vi "GetImageFileMachineVersion.vi"(8 "error in":errorcluster, 11 "dll Path":path) -> (0 "error out":errorcluster, 2 "bitness":enum16{"unknown", "32", "64"}(ring), 3 "path":path)   [LabVIEW 2017]
doc: "This VI can will read the PE Header to read the Machine type (x86 or x64)"
uses:
  <vilib>/ErrorRing/Error Ring.xnode
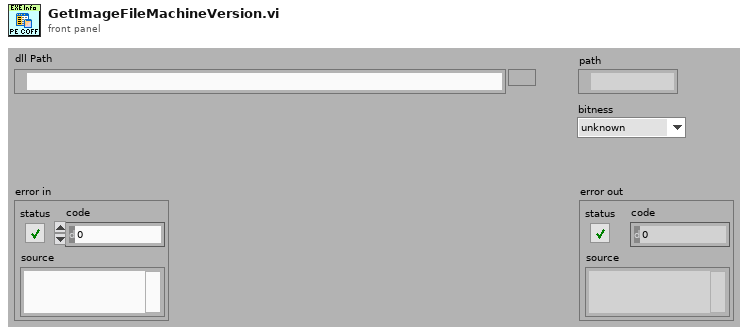
[diagram p1: front panel]
types:
  T1 = enum16{"open", "replace", "create", "open or create", "replace or create", "replace or create with confirmation"}
  T2 = enum16{"big-endian, network order", "native, host order", "little-endian"}
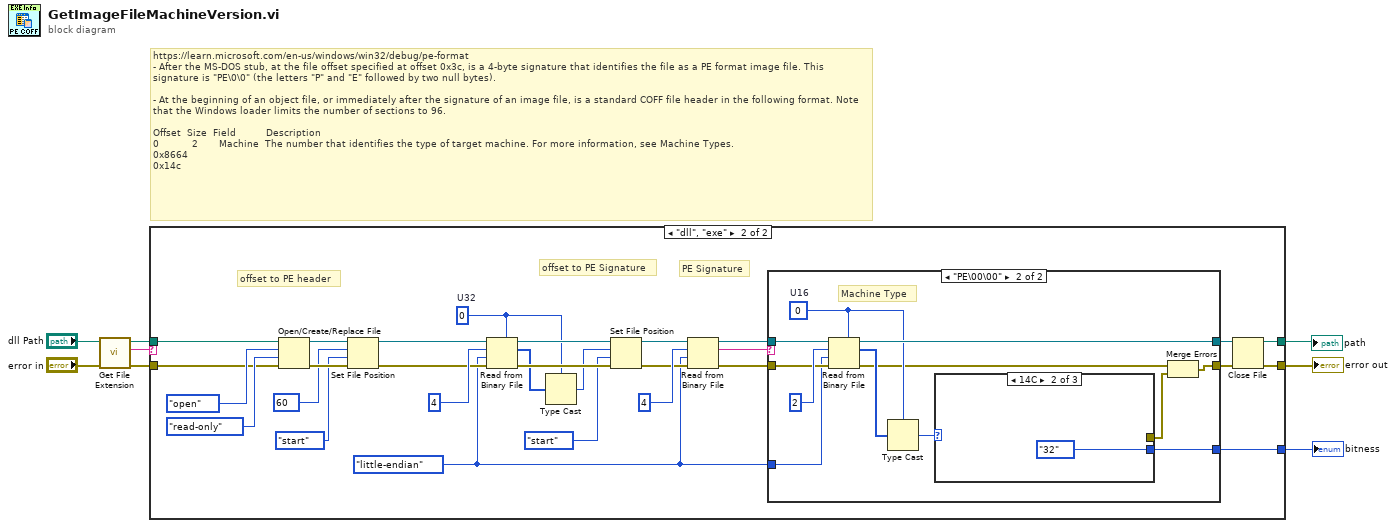
[diagram p0: block diagram]
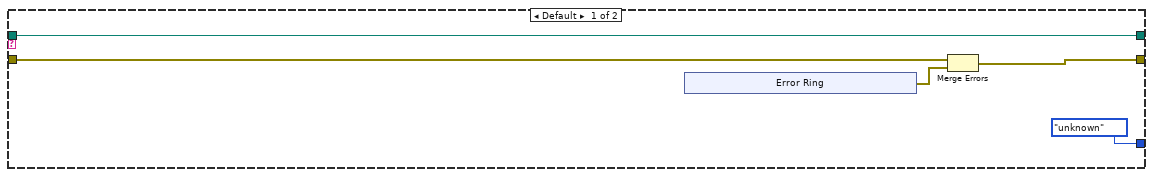
[diagram p2: hidden frame]
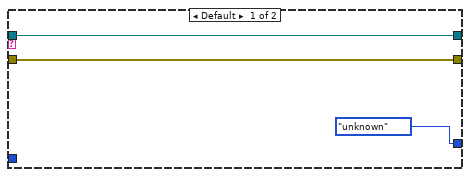
[diagram p3: hidden frame]
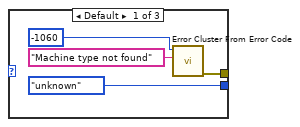
[diagram p4: hidden frame]
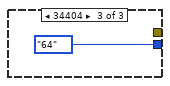
[diagram p5: hidden frame]
diagram:
  # "https://learn.microsoft.com/en-us/windows/win32/debug/pe-format\n- After the MS-DOS stub, at the file offset specified at offset 0x3c, is a 4-byte signature that identifies the file as a PE format image file. This signature is \"PE\\0\\0\" (the letters \"P\" and \"E\" followed by two null bytes).\n\n- At the beginning of an object file, or immediately after the signature of an image file, is a standard COFF file header in the following format. Note that the Windows loader limits the number of sections to 96.\n\nOffset \tSize \tField \t        Description\n0\t          2\t      Machine\t The number that identifies the type of target machine. For more information, see Machine Types. \n0x8664 \n0x14c"
  n1 = call <vilib>:"Get File Extension.vi"("error in (no error)"="error in", "file"="dll Path") -> ("error out"=w6:errorcluster, "lowercase file extension"=w4:string, "dup file"=w5:path)  [unwired: 5 in, 2 out]
  n2 = case shown="\"dll\", \"exe\"" w4 {
    tunnel: w6 -> [w13 w26]
    tunnel: w5 -> [w9 w25]
    tunnel: [w11 w22] -> w3
    tunnel: [enum16{"unknown", "32", "64"}."unknown" ("bitness") w20] -> w2
    tunnel: [w9 w18] -> w1
    frame Default {
      n3 = xnode "Error Ring"() -> ("error out"=w12:errorcluster)
      n4 = Merge Errors(w13, w12) -> (w11:errorcluster)
    }
    frame "dll", "exe" {
      w19 = u32 0  # U32
      w27 = T2."little-endian" ("byte order (0:big-endian, network order)")
      # "PE Signature"
      # "offset to PE Signature"
      # "offset to PE header"
      n5 = Open/Create/Replace File(file path (use dialog)=w25, error in=w26, operation (0:open)=T1."open", access (0:read/write)=enum16{"read/write", "read-only", "write-only"}."read-only") -> (refnum out=w45:refnum<file>, error out=w44:errorcluster)  [unwired: 2 in, 1 out]
      n6 = Set File Position(offset (in bytes) (0)=i64 60, refnum=w45, from (0:start)=enum16{"start", "end", "current"}."start", error in=w44) -> (refnum out=w41:refnum<file>, error out=w40:errorcluster)
      n7 = Read from Binary File(5:w19, 8:w40, 9:w27, 10:4 ("count (1)"), 11:w41) -> (0:w38:errorcluster, 2:w33:u32[], 3:w39:refnum<file>)  [unwired: 1 in, 1 out]
      n8 = Type Cast(type=w19, x=w33) -> (*(type *) &x=w35:u32)
      n9 = Set File Position(offset (in bytes) (0)=w35, refnum=w39, from (0:start)=enum16{"start", "end", "current"}."start", error in=w38) -> (refnum out=w31:refnum<file>, error out=w30:errorcluster)
      n10 = Read from Binary File(8:w30, 9:w27, 10:4 ("count (1)"), 11:w31) -> (0:w28:errorcluster, 2:w21:string, 3:w29:refnum<file>)  [unwired: 2 in, 1 out]
      n11 = case shown="\"PE\\00\\00\"" w21 {
        tunnel: [w48 w61] -> w23
        tunnel: [w49 w53] -> w24
        tunnel: w29 -> [w48 w59]
        tunnel: w28 -> [w49 w58]
        tunnel: w27 -> [_ w57]
        tunnel: [enum16{"unknown", "32", "64"}."unknown" ("bitness") w50] -> w20
        frame Default {
        }
        frame "PE\u0000\u0000" {
          w55 = u16 0  # U16
          # "Machine Type"
          n12 = Read from Binary File(5:w55, 8:w58, 9:w57, 10:2 ("count (1)"), 11:w59) -> (0:w51:errorcluster, 2:w56:u16[], 3:w61:refnum<file>)  [unwired: 1 in, 1 out]
          n13 = Type Cast(type=w55, x=w56) -> (*(type *) &x=w54:u16)
          n14 = case shown="14C" w54 {
            tunnel: [w65 _ _] -> w52
            tunnel: [enum16{"unknown", "32", "64"}."unknown" ("bitness") enum16{"unknown", "32", "64"}."32" ("bitness") enum16{"unknown", "32", "64"}."64" ("bitness")] -> w50
            frame Default {
              n15 = call <vilib>:"Error Cluster From Error Code.vi"("error message (\"\")"="Machine type not found" ("error message (\"\")"), "error code (0)"=-1060) -> ("error out"=w65:errorcluster)  [unwired: 7 in]
            }
            frame 332 {
            }
            frame 34404 {
            }
          }
          n16 = Merge Errors(w51, w52) -> (w53:errorcluster)
        }
      }
      n17 = Close File(refnum=w23, error in=w24) -> (path=w18:path, error out=w22:errorcluster)
    }
  }
  "error out" <- w3
  "bitness" <- w2
  "path" <- w1
